vi "Async Reply.vi"(7 "Sender":refnum<class "Sender.lvclass">, 9 "Is Priority":bool, 10 "Msg":refnum<class "Msg.lvclass">, 11 "Base Actor in":refnum<class "Base Actor.lvclass">) -> (3 "Base Actor out":refnum<class "Base Actor.lvclass">)   [LabVIEW 2020, in "jettl.lvlib" / "Actor.lvlib" / "Base Actor.lvclass"]
uses:
  Base Actor.lvclass
  Sender/Sender/Sender.lvclass
  Msg/Msg.lvclass
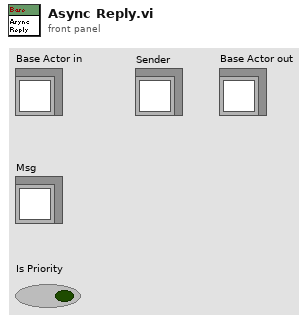
[diagram p1: front panel]
types:
  T1 = typedef "jettl.lvlib/Sender.lvlib/Relation.ctl" = enum16{"Self", "Creator", "Created"}
  T2 = typedef "jettl.lvlib/Actor.lvlib/Attributes.ctl" = cluster{"Alias":string, "Address":refnum<user-event>, "Implemented Msgs":T3, "Path":path}
  T3 = typedef "jettl.lvlib/Actor.lvlib/Implemented Msgs.ctl" = set{refnum<class "Msg.lvclass">}
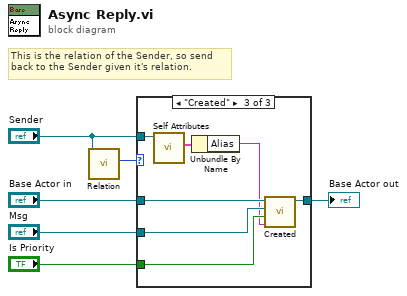
[diagram p0: block diagram]
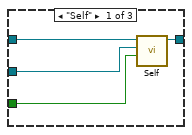
[diagram p2: hidden frame]
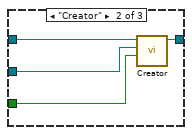
[diagram p3: hidden frame]
diagram:
  # "This is the relation of the Sender, so send back to the Sender given it's relation."
  n1 = call-dynamic "Relation.vi"("Sender in"="Sender") -> ("Relation"=w6:T1)  [unwired: 10 in]
  n2 = case shown="\"Created\"" w6 {
    tunnel: [w9 w13 w20] -> w5
    tunnel: "Base Actor in" -> [w10 w14 w21]
    tunnel: "Msg" -> [w8 w12 w19]
    tunnel: "Is Priority" -> [w7 w11 w18]
    tunnel: "Sender" -> [_ _ w17]
    frame "Self" {
      n3 = call-dynamic "Self.vi"("Is Priority"=w7, "Msg"=w8, "Base Actor in"=w10) -> ("Base Actor out"=w9:refnum<class "Base Actor.lvclass">)  [unwired: 8 in]
    }
    frame "Creator" {
      n4 = call-dynamic "Creator.vi"("Is Priority"=w11, "Msg"=w12, "Base Actor in"=w14) -> ("Base Actor out"=w13:refnum<class "Base Actor.lvclass">)  [unwired: 8 in]
    }
    frame "Created" {
      n5 = call-dynamic "Self Attributes.vi"("Sender in"=w17) -> ("Self Attributes"=w16:T2)  [unwired: 10 in]
      n6 = Unbundle By Name(w16) -> ("Alias"=w15:string)
      n7 = call-dynamic "Created.vi"("Created Alias"=w15, "Is Priority"=w18, "Msg"=w19, "Base Actor in"=w21) -> ("Base Actor out"=w20:refnum<class "Base Actor.lvclass">)  [unwired: 7 in]
    }
  }
  "Base Actor out" <- w5
